vi "Build Nav HTTP.vi"(7 "TemplateService":refnum<class "TemplateService.lvclass">, 11 "VolatusVariableResolver in":refnum<class "VolatusVariableResolver.lvclass">) -> (2 "Value":refnum<class "Value Tree.lvclass">)   [LabVIEW 2020, in "Volatus.lvlib" / "VolatusVariableResolver.lvclass"]
uses:
  VolatusVariableResolver.lvclass
  VolatusVariableResolver.lvclass/VolatusVariableResolver.ctl
  21439c05-09ab-46e8-8256-af0f678bac29.vi
  Nav Route/Nav Route.lvclass
  lv-http-server/HTTP Server/Value Tree/Value Tree.lvclass
  lv-http-server/HTTP Server/Value Tree/Local Type.ctl
  lv-http-server/HTTP Server/TemplateService/TemplateService.lvclass
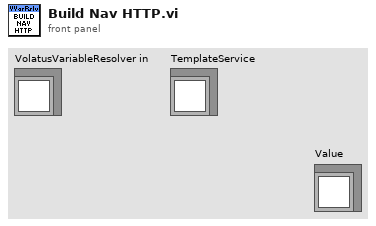
[diagram p1: front panel]
types:
  T1 = typedef "HTTP Server.lvlib/Value Tree.lvclass/Local Type.ctl" = enum16{"Scalar", "Object", "Array"}
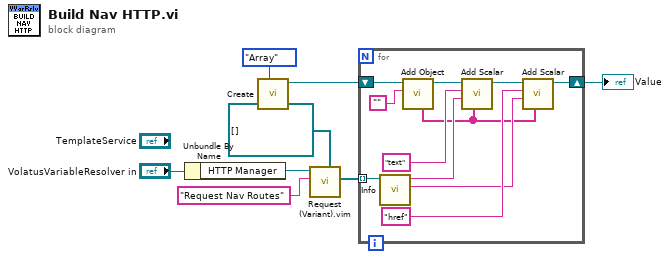
[diagram p0: block diagram]
diagram:
  n1 = Unbundle By Name("VolatusVariableResolver in") -> ("HTTP Manager"=w8:refnum<class "MessageQ.lvclass">)
  n2 = call "Create.vi"("Root Type (Scalar)"=Local_Type."Array") -> ("Value Tree out"=w2:refnum<class "Value Tree.lvclass">)  [unwired: 10 in]
  n3 = call "Request (Variant).vim"("Type"=refnum<class "Nav Route.lvclass">[] [], "ID"="Request Nav Routes", "MessageQ in"=w8) -> ("Value"=w4:refnum<class "Nav Route.lvclass">[])  [unwired: 6 in, 2 out]
  n4 = for {
    tunnel: w4 -> [w19] mode=indexing
    shift-right: [w9] -> w1
    shift-left: w2 -> [w12]
    n5 = call "Info.vi"("Nav Route in"=w19) -> ("Path"=w14:string, "Label"=w17:string)  [unwired: 7 in, 2 out]
    n6 = call "Add Object.vi"("Name"="", "TemplateLocals in"=w12) -> ("TemplateLocals out"=w11:refnum<class "Value Tree.lvclass">, "Hierarchy"=w10:string[])  [unwired: 7 in, 1 out]
    n7 = call "Add Scalar.vi"("Parent (None)"=w10, "Value"=w17, "Name"="text" ("key"), "TemplateLocals in"=w11) -> ("TemplateLocals out"=w16:refnum<class "Value Tree.lvclass">)  [unwired: 5 in, 2 out]
    n8 = call "Add Scalar.vi"("Parent (None)"=w10, "Value"=w14, "Name"="href" ("key"), "TemplateLocals in"=w16) -> ("TemplateLocals out"=w9:refnum<class "Value Tree.lvclass">)  [unwired: 5 in, 2 out]
  }
  "Value" <- w1
